vi "Create Deinterleave Sample Buffer.vi"(0 "device session in":refnum<class "Device Session.lvclass">, 5 "read size in samples":u32, 11 "error in":errorcluster) -> (4 "device session out":refnum<class "Device Session.lvclass">, 6 "buffer":i16[][](array[numeric]), 15 "error out":errorcluster)   [LabVIEW 2015, in "Device Session.lvclass"]
doc: "Takes in the number of samples fetched and creates a two-dimensional buffer to hold the fetched data after it has been deinterleaved.\n\n<B>Input Parameters</B>\n\n<B>device session in</B> is a reference to the session containing sessions to all instrument design libraries used in this sample project. This parameter is obtained from the 'Open Session' VI.\n\n<B>read size in samples</B> specifies the number of samples per channel fetched.\n\n<B>error in</B> describes error conditions that occur before this node runs. This input provides standard 'error in' functionality.\n\n<B>Output Parameters</B>\n\n<B>device session out</B> passes a reference to the session to the next VI.\n\n<B>buffer</B> returns a two-dimensional array with dimensional lengths of samples per channel and number of channels streamed.\n\n<B>error out</B> contains error information. This output provides standard 'error out' functionality."
uses:
  Device Session.lvclass
  Device Session.lvclass/Device Session.ctl
  <instrlib>/_niInstr/Data Manipulation/v1/Host/Private/Reshape I162D.vi
  <instrlib>/_niInstr/Data Manipulation/v1/Host/niInstr Data Manipulation v1 Host.lvlib
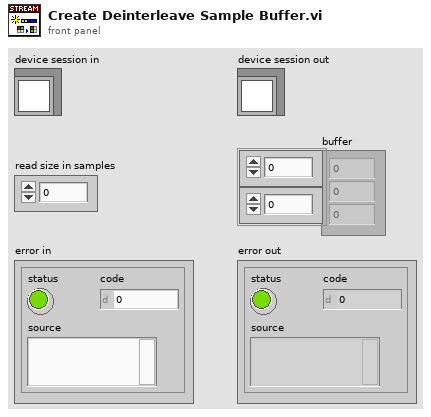
[diagram p1: front panel]
types:
  T1 = typedef "Device Session.lvclass/Device Session Object.ctl" = cluster{"ni5171R FPGA Reference":T2, "niHSAI config":refnum<class "niHSAI Config v1 Host.lvclass">, "configured scaling coefficients":cluster{"gain":dbl, "offset":dbl}[], "number of channels to stream":u8, "selected acq channels":bool[], "number of channels":u32, "actual channel configuration":T3[], "configured channels":bool[], "sample clock rate (Hz)":dbl}
  T2 = typedef "Device Session.lvclass/FPGA Refnum.ctl" = refnum<k20>
  T3 = typedef "niHSAI Types v1 Host.lvlib/Channel Configuration.ctl" = cluster{"channel":u32, "coupling":T4, "impedance":T5, "bandwidth":T6, "vertical range":dbl, "vertical offset":dbl}
  T4 = typedef "niHSAI Types v1 Host.lvlib/Coupling.ctl" = enum8{"Default", "DC", "AC"}
  T5 = typedef "niHSAI Types v1 Host.lvlib/Impedance.ctl" = enum8{"Default", "1 mega ohm", "50 ohm"}
  T6 = typedef "niHSAI Types v1 Host.lvlib/Bandwidth.ctl" = enum8{"Default", "Full Bandwidth", "Anti-alias Filter"}
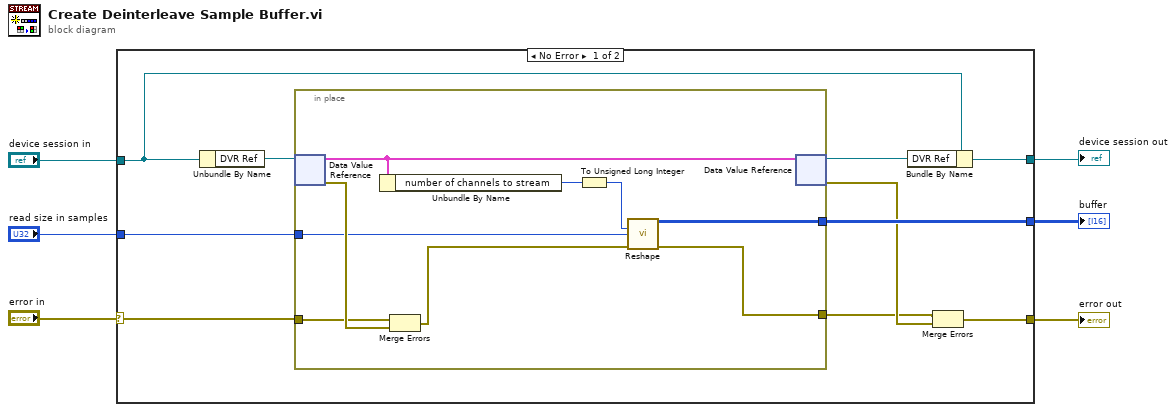
[diagram p0: block diagram]
diagram:
  n1 = case shown="No Error" "error in" {
    selector: "error in" -> [w16 w27]
    tunnel: "device session in" -> [w13 w26]
    tunnel: [w12 w26] -> w5
    tunnel: [w11 w27] -> w2
    tunnel: "read size in samples" -> [w10 _]
    tunnel: [w9 _] -> w1
    frame No Error {
      n2 = Unbundle By Name(w13) -> ("DVR Ref"=w15:refnum<data-value>)
      n3 = in-place {
        in-place-border: w16 -> [w23]
        in-place-border: [w20] -> w7
        in-place-border: w10 -> [w22]
        in-place-border: [w19] -> w9
        n4 = in-place-dvr #1(w15) -> (w25:T1, w24:errorcluster)
        n5 = Unbundle By Name(w25) -> ("number of channels to stream"=w18:u8)
        n6 = Merge Errors(w23, w24) -> (w21:errorcluster)
        n7 = To Unsigned Long Integer(number=w18) -> (unsigned 32bit integer=w17:u32)
        n8 = call-poly <instrlib>:"Reshape.vi"("dimension size 0"=w17, "dimension size 1"=w22, "error in"=w21) -> ("reshaped array"=w19:i16[][], "error out"=w20:errorcluster)  [unwired: 10 in, 1 out]
        n9 = in-place-dvr #1(w25) -> (w14:refnum<data-value>, w8:errorcluster)
      }
      n10 = Bundle By Name(cluster=w13, "DVR Ref"=w14) -> (w12:refnum<class "Device Session.lvclass">)
      n11 = Merge Errors(w7, w8) -> (w11:errorcluster)
    }
    frame Error {
    }
  }
  "buffer" <- w1
  "error out" <- w2
  "device session out" <- w5
